vi "CalibrationManagementDemo.vi"() -> ()   [LabVIEW 2019]
uses:
  TypeDef/SlugExpiration.ctl
  ByteQXAPIBase/ByteQXAPIBase.lvclass
  TypeDef/CalibrationStates.ctl
  ByteQXAPIBase/FetchCalibration/Converted_Slug_Cluster.ctl
  ByteQXAPIBase/Instruments/Instrument.ctl
  ByteQXAPIBase/CalibrationMeasurements/CalibMeasure.ctl
  aa47c742-c095-4670-bf1f-6b28e4309cef.vi
  <vilib>/numeric/Random Number (Range) I64.vi
  <vilib>/Array/Sort 2D Array - Pop Stack.vi
  <vilib>/Array/Sort 2D Array - Push Stack.vi
  <vilib>/numeric/sub_Random U32.vi
panel:
  in  "Exit":bool
  out "Calibrations":string
  out "Status":string
  out "Calibration n.":string
  in  "Cancel":bool
  in  "Approvation":bool
  in  "Avanti":bool
  in  "Repeat":bool
  out "Outcome":string
  out "Measured value":dbl
  out "Reference value":dbl
  out "Waveform Chart":i64(graph)
  in  "Start Calibration":bool
  in  "Next":bool
  in  "Previus":bool
  out "Calibration n.":string
  in  "Filter":enum16{"All", "Expired", "Not Expired"}(ring)
  in  "Slug list":T1[](array[typedef])
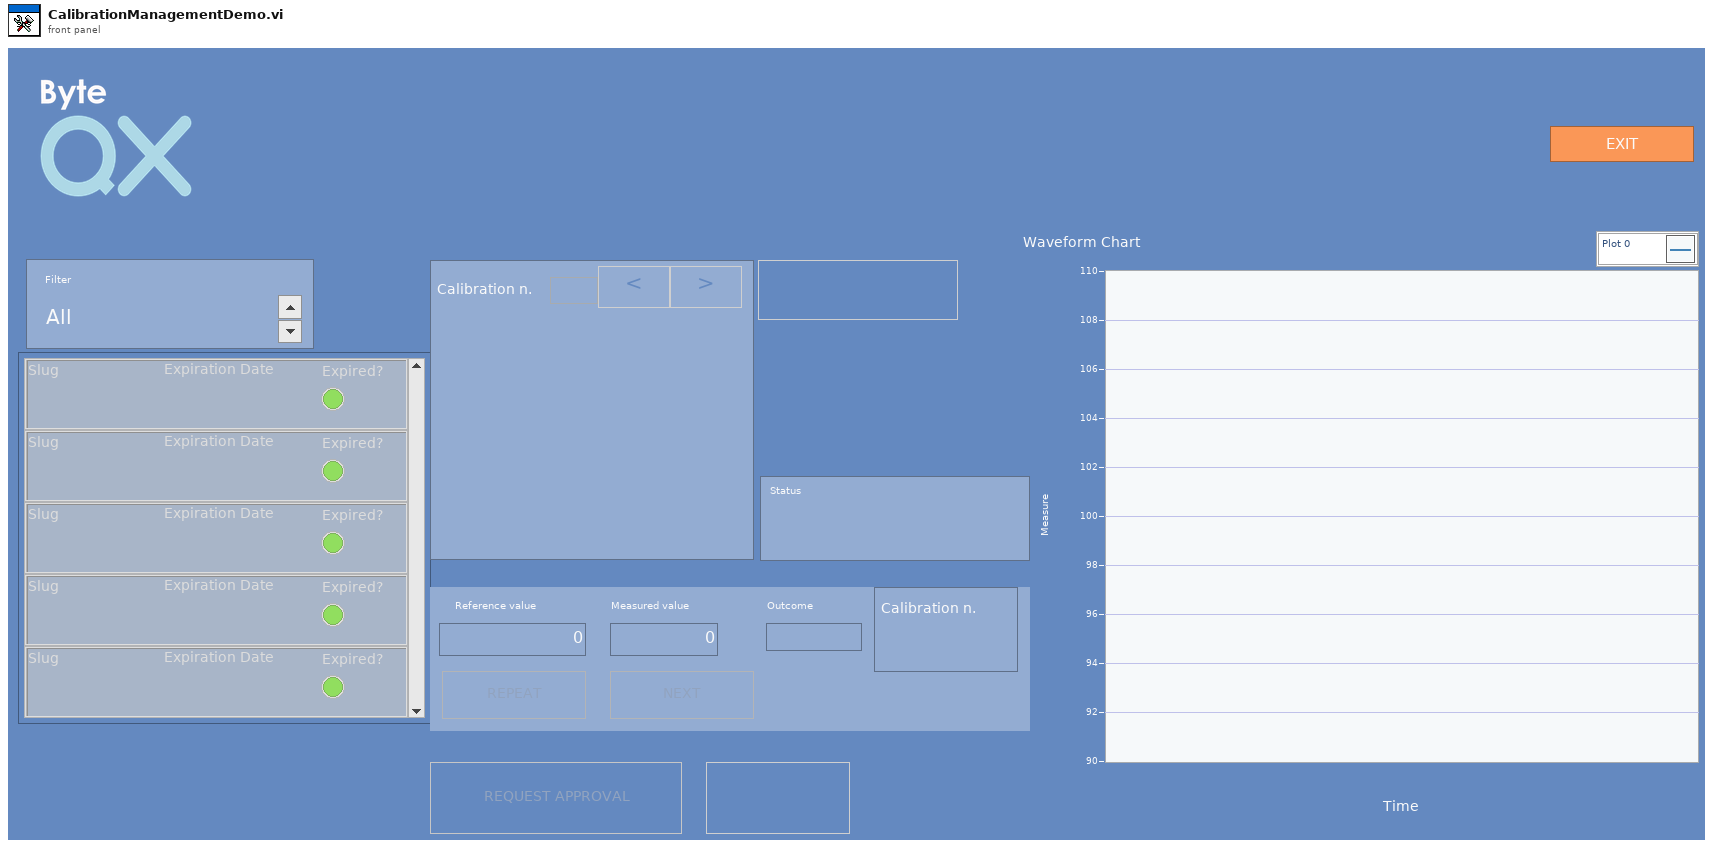
[diagram p1: front panel]
types:
  T1 = typedef "SlugExpiration.ctl" = cluster{"Slug":string, "Expiration Date":string, "Expired?":bool, "Id":i32, "active":bool, "Color Box":u32}
  T2 = typedef "CalibrationStates.ctl" = enum16{"Init", "Idle", "GetInstruments", "Fetch", "GetCalibrations", "CheckTotalMisurations", "StartCalibration", "ManageCalibration", "AllowApprove", "Approve"}
  T3 = typedef "ByteQXWebAPI.lvlib/ByteQXAPIBase.lvclass/CalibMeasure.ctl" = cluster{"controls":cluster{"id":u16, "descrizione":string, "numero_misure_necessarie":u16, "riferimento_obiettivo":dbl, "mpe_max":dbl, "mpe_min":dbl, "deviazione_standard":dbl, "incertezza":dbl, "numero_misure_effettuate":u32, "temperatura_c":dbl, "umidita":dbl, "strumento_riferimento":cluster{"id":u16, "nome":string}[]}[]}
  T4 = typedef "ByteQXWebAPI.lvlib/ByteQXAPIBase.lvclass/Instrument.ctl" = cluster{"id":i32, "slug":string, "stabilimento":cluster{"id":dbl}, "categoria":cluster{"id":dbl}, "tipologia_di_visualizzazione":cluster{"id":dbl}, "stato":cluster{"id":dbl}, "descrizione":string, "costruttore":string, "matricola":string, "data_registrazione":string, "intervallo_di_taratura_mesi":dbl, "reparto":string, "campo_misura":string, "risoluzione":dbl, "responsabile_strumento":string, "classe_di_precisione":string, "classificazione":string, "appunti":string, "manuale":string, "foto":string, "riferimento":bool, "qr_hashcode":string, "costo_euro":dbl}
  T5 = typedef "ByteQXWebAPI.lvlib/ByteQXAPIBase.lvclass/Converted_Slug_Cluster.ctl" = cluster{"id":u32, "instrument":string, "name":string, "date":timestamp}
  T6 = cluster{"Outcome":refnum<vi>, "Avanti":refnum<vi>, "Repeat":refnum<vi>, "Slug list":refnum<vi>, "Start Calibration":refnum<vi>, "Avanti":refnum<vi>, "Cancel":refnum<vi>, "Approvation":refnum<vi>}
  T7 = cluster{"ByteQXAPIBase in":refnum<class "ByteQXAPIBase.lvclass">, "Instruments_Slug":string[], "All_Instruments_Cals":T5[], "All_Instruments":T4[], "Slug list All":T1[], "Calibrations":T3, "Selected Slug":i32, "Misurazioni":string, "Misurazioni index":i32, "Next State":T2, "Waveform Chart":refnum<vi>, "New Val":dbl, "Id Failed":u32, "Failed?":bool, "Cal Index":i32, "Misurazioni n":string, "Stato":string, "Esito":string, "Misure effettuate":i32, "Calibrations":string}
  T8 = typedef "SlugExpiration1.ctl" = cluster{"Slug":string, "Expiration Date":string, "Expired?":bool, "Id":i32, "active":bool, "Color Box":u32}
  T9 = cluster{"id":u16, "descrizione":string, "numero_misure_necessarie":u16, "riferimento_obiettivo":dbl, "mpe_max":dbl, "mpe_min":dbl, "deviazione_standard":dbl, "incertezza":dbl, "numero_misure_effettuate":u32, "temperatura_c":dbl, "umidita":dbl, "strumento_riferimento":cluster{"id":u16, "nome":string}[]}[]
  T10 = cluster{"id":u16, "descrizione":string, "numero_misure_necessarie":u16, "riferimento_obiettivo":dbl, "mpe_max":dbl, "mpe_min":dbl, "deviazione_standard":dbl, "incertezza":dbl, "numero_misure_effettuate":u32, "temperatura_c":dbl, "umidita":dbl, "strumento_riferimento":cluster{"id":u16, "nome":string}[]}
  T11 = typedef "ByteQXWebAPI.lvlib/ByteQXAPIBase.lvclass/MeasurementResData.ctl" = cluster{"id":i32, "gruppo_misurazione":cluster{"id":i32}, "misura_strumento":dbl, "misura_riferimento":dbl, "is_correct":bool}
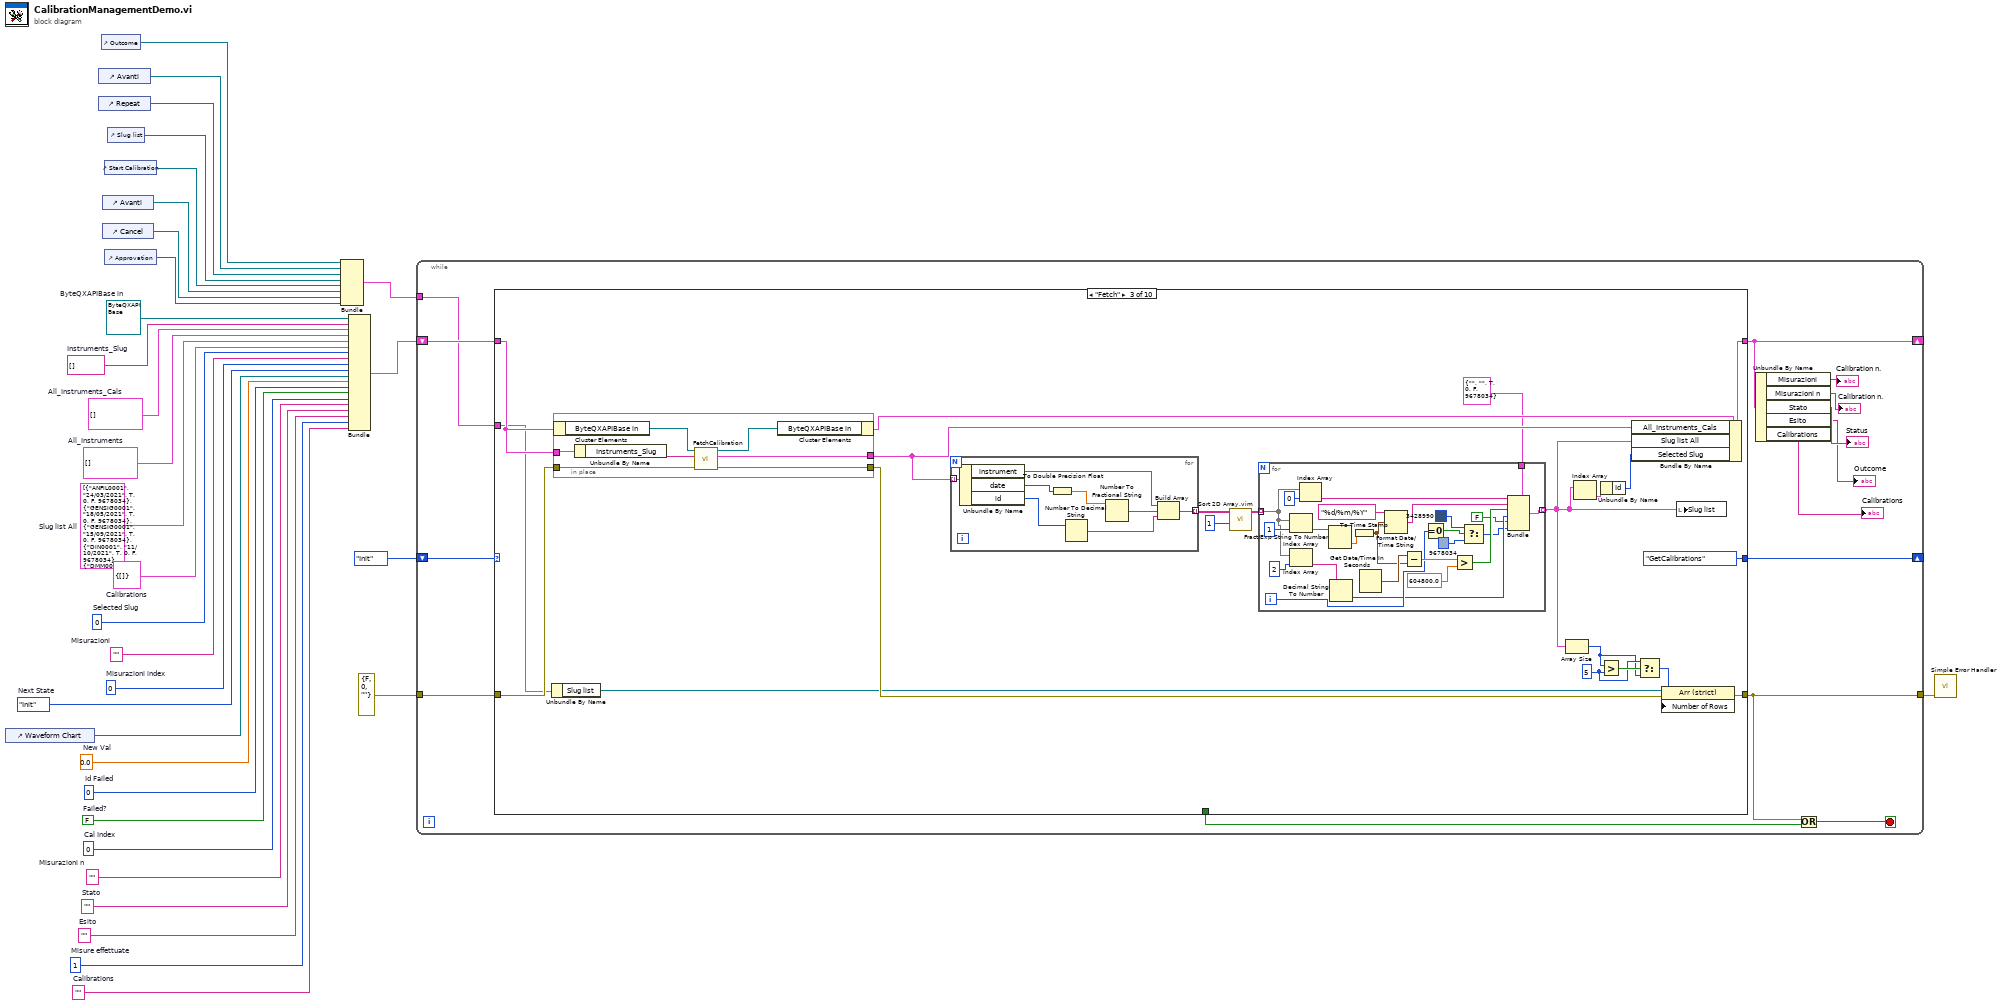
[diagram p0: block diagram]
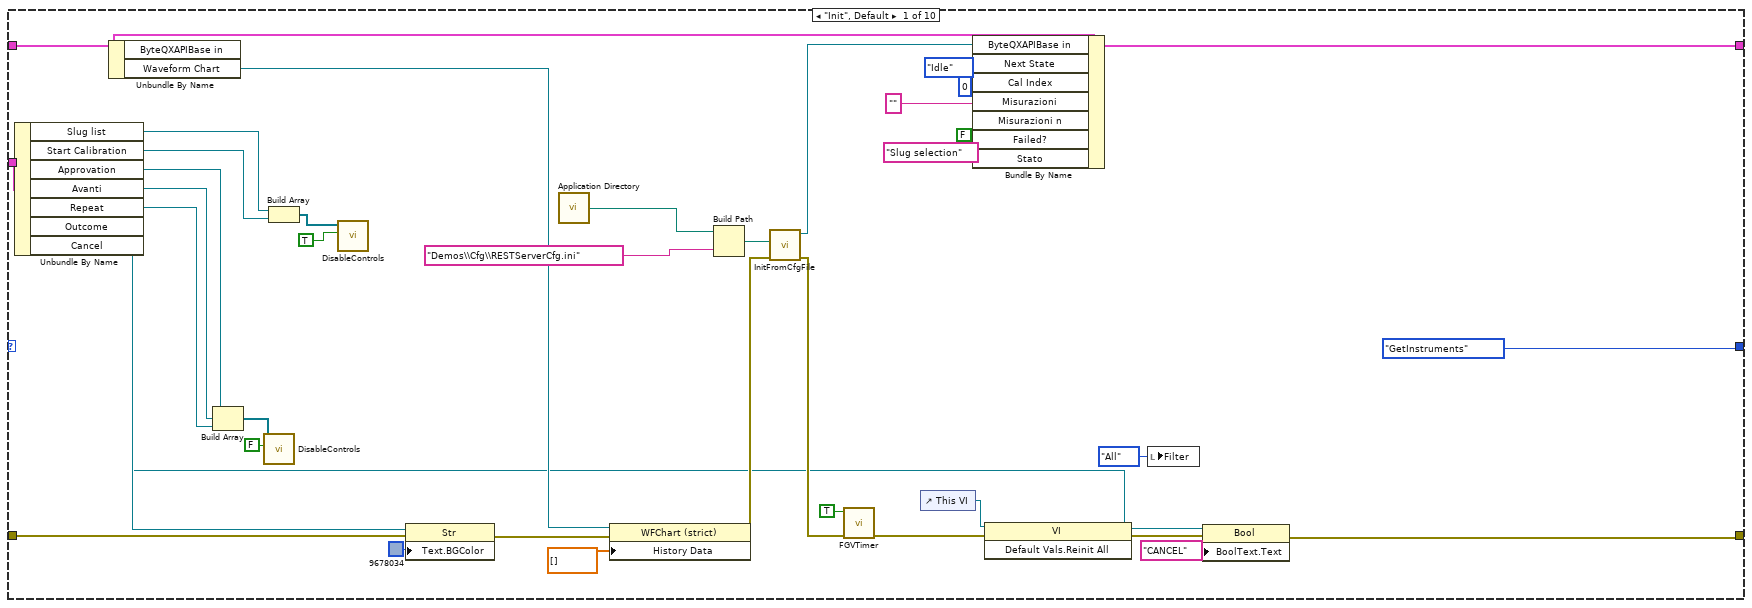
[diagram p2: hidden frame]
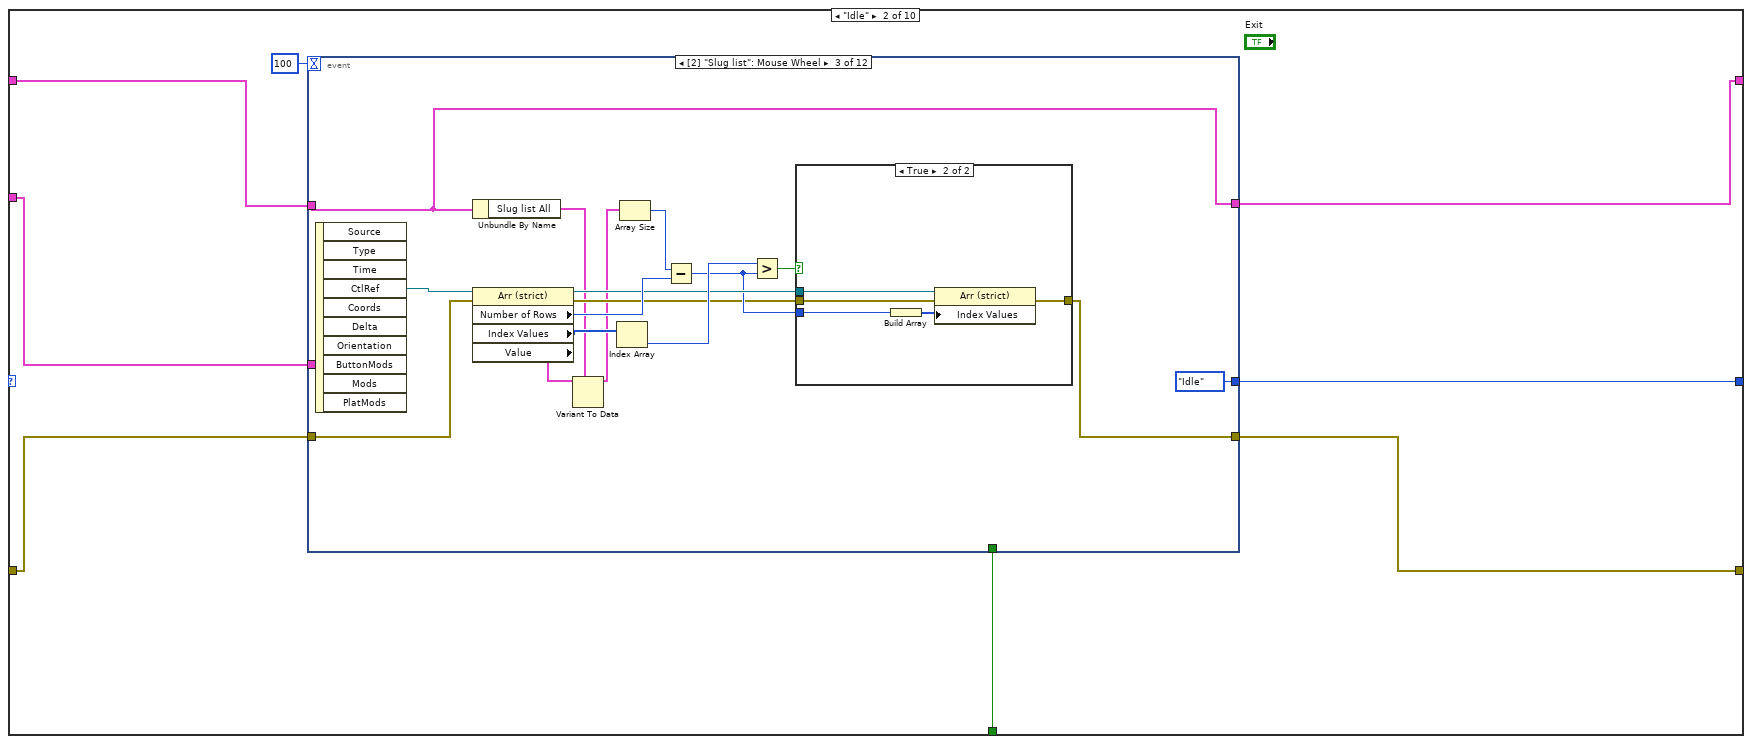
[diagram p3: hidden frame]
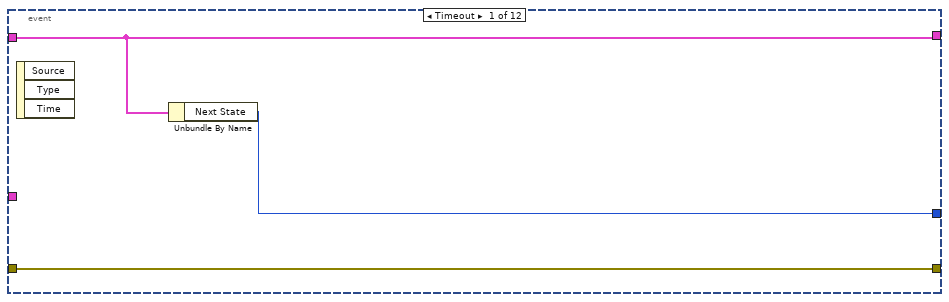
[diagram p4: hidden frame]
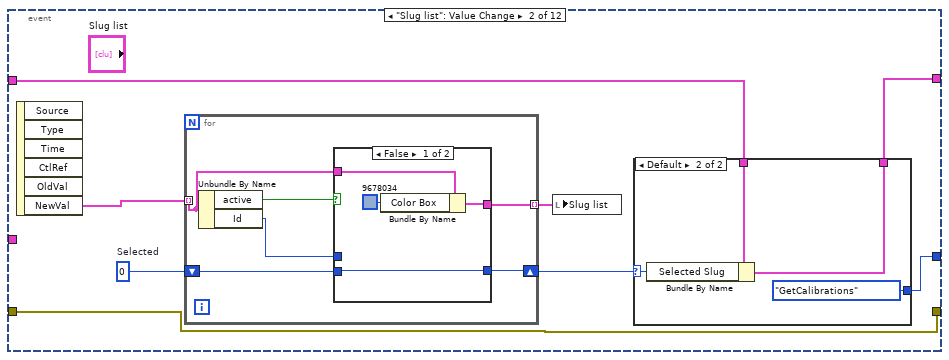
[diagram p5: hidden frame]
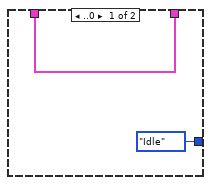
[diagram p6: hidden frame]
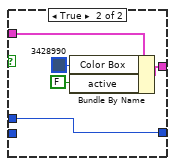
[diagram p7: hidden frame]
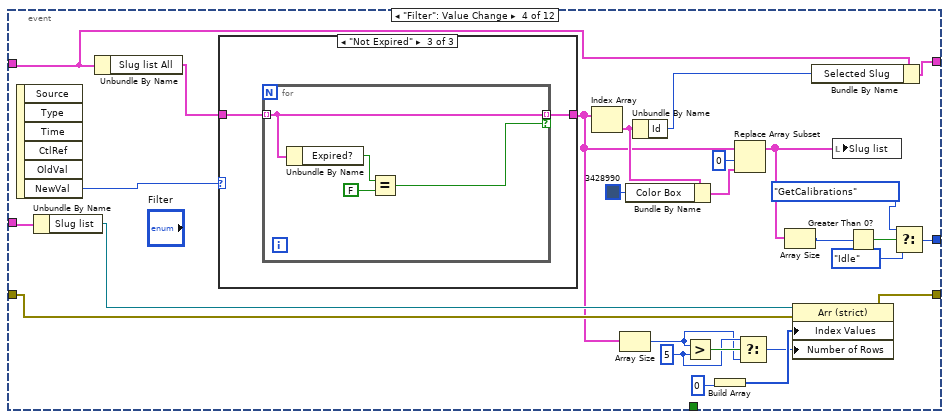
[diagram p9: hidden frame]
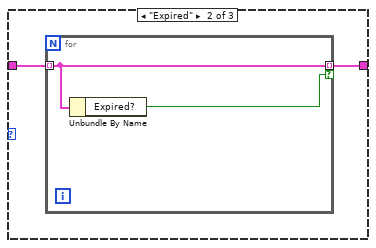
[diagram p11: hidden frame]
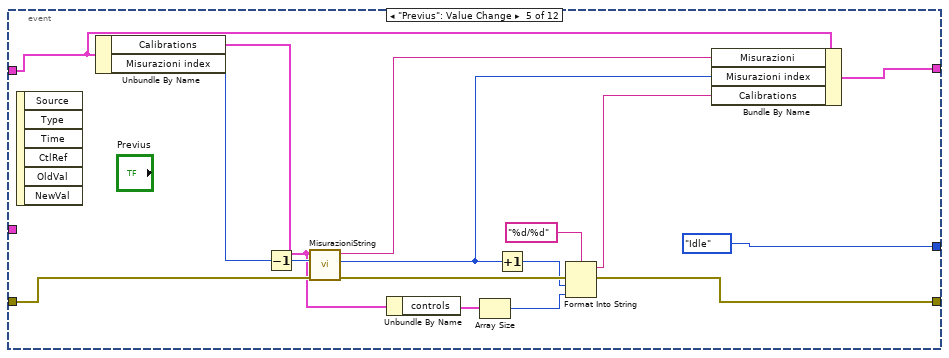
[diagram p12: hidden frame]
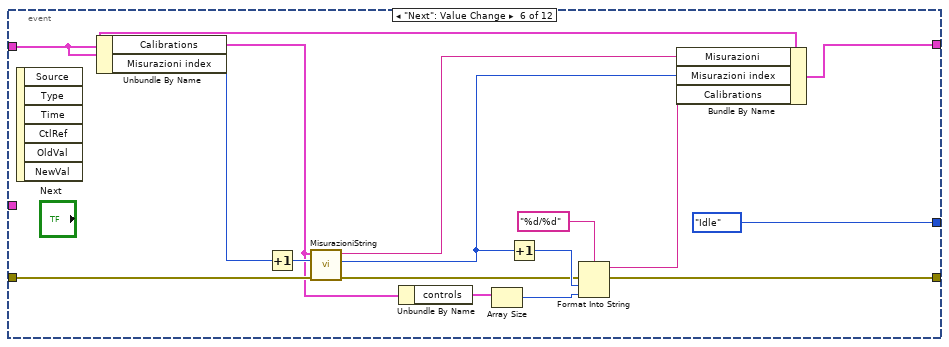
[diagram p13: hidden frame]
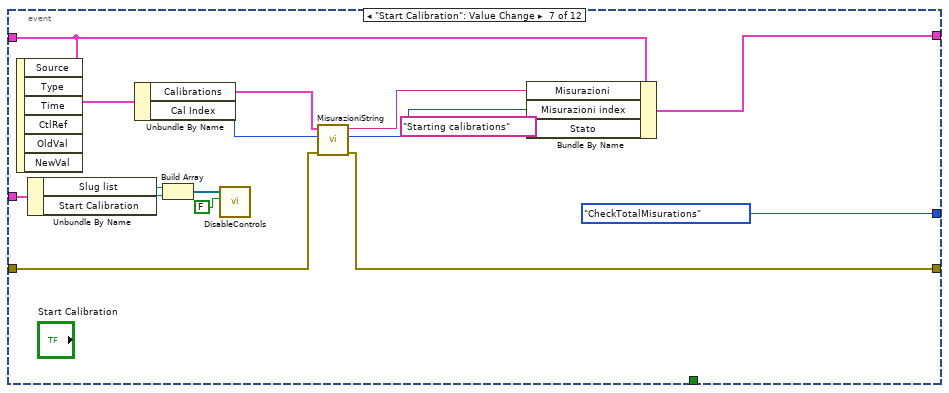
[diagram p14: hidden frame]
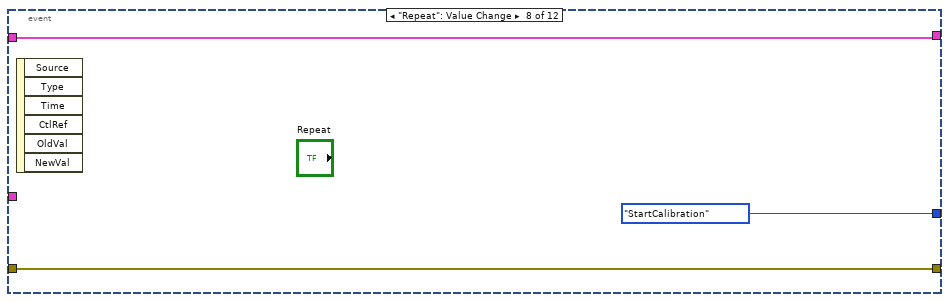
[diagram p15: hidden frame]
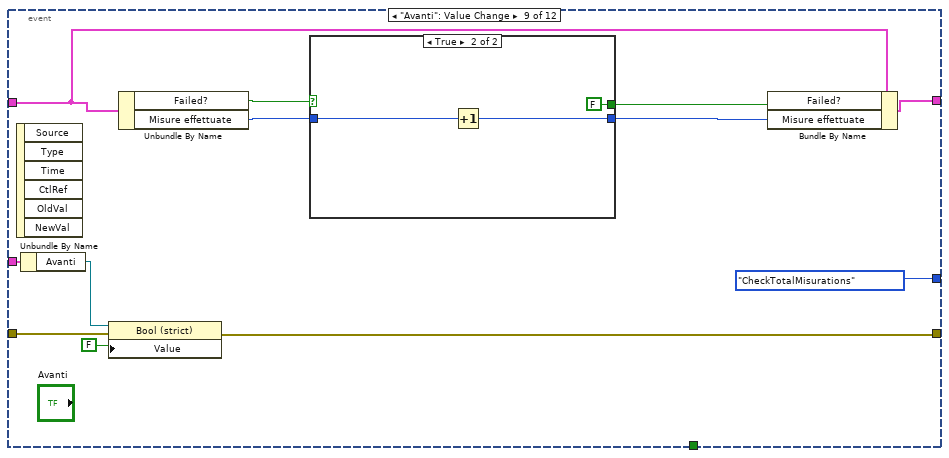
[diagram p16: hidden frame]
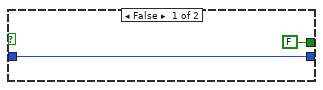
[diagram p17: hidden frame]
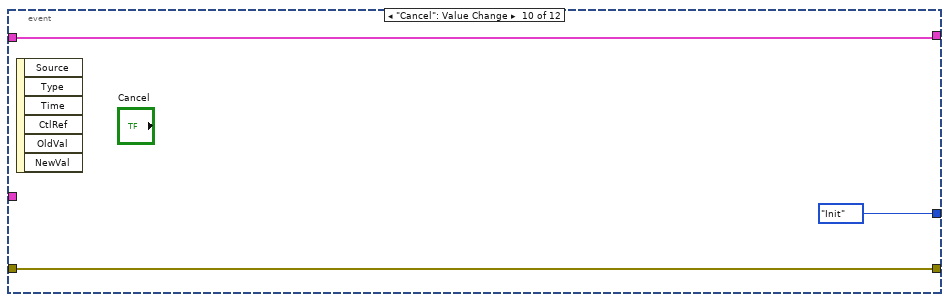
[diagram p18: hidden frame]
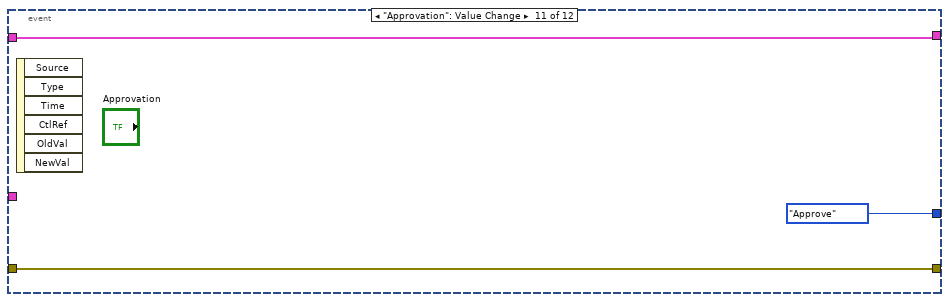
[diagram p19: hidden frame]
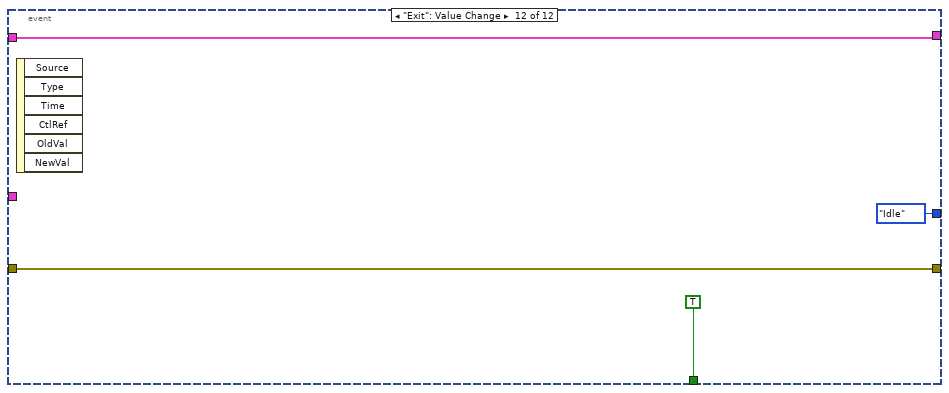
[diagram p20: hidden frame]
diagram:
  w2 = ""  # Calibrations
  w3 = 1  # Misure effettuate
  w5 = ""  # Esito
  w6 = ""  # Stato
  w11 = ""  # Misurazioni n
  w16 = 0  # Cal Index
  w17 = FALSE  # Failed?
  w18 = u32 0  # Id Failed
  w19 = 0.0  # New Val
  w21 = CalibrationStates."Init"  # Next State
  w22 = 0  # Misurazioni index
  w23 = ""  # Misurazioni
  w24 = T1[] [{"Slug"="ANFIL0001", "Expiration Date"="24/03/2021", "Expired?"=TRUE, "Id"=0, "active"=FALSE, "Color Box"=9678034}, {"Slug"="GENSIG0001", "Expiration Date"="18/05/2021", "Expired?"=TRUE, "Id"=0, "active"=FALSE, "Color Box"=9678034}, {"Slug"="GENSIG0001", "Expiration Date"="15/09/2021", "Expired?"=TRUE, "Id"=0, "active"=FALSE, "Color Box"=9678034}, {"Slug"="DIN0001", "Expiration Date"="11/10/2021", "Expired?"=TRUE, "Id"=0, "active"=FALSE, "Color Box"=9678034}, {"Slug"="DMM0002", "Expiration Date"="20/10/2021", "Expired?"=TRUE, "Id"=0, "active"=FALSE, "Color Box"=9678034}, {"Slug"="COMP0001", "Expiration Date"="01/12/2021", "Expired?"=TRUE, "Id"=0, "active"=FALSE, "Color Box"=9678034}, {"Slug"="TORS0002", "Expiration Date"="06/12/2021", "Expired?"=TRUE, "Id"=0, "active"=FALSE, "Color Box"=9678034}, {"Slug"="CDIND0001", "Expiration Date"="04/03/2022", "Expired?"=TRUE, "Id"=0, "active"=FALSE, "Color Box"=9678034}, {"Slug"="CALI0004", "Expiration Date"="11/03/2022", "Expired?"=TRUE, "Id"=0, "active"=FALSE, "Color Box"=9678034}, {"Slug"="CALI0001", "Expiration Date"="10/05/2022", "Expired?"=TRUE, "Id"=0, "active"=FALSE, "Color Box"=9678034}, {"Slug"="CALI0012", "Expiration Date"="10/05/2022", "Expired?"=TRUE, "Id"=0, "active"=FALSE, "Color Box"=9678034}, {"Slug"="CALI0011", "Expiration Date"="11/05/2022", "Expired?"=TRUE, "Id"=0, "active"=FALSE, "Color Box"=9678034}, {"Slug"="CALI0014", "Expiration Date"="04/07/2022", "Expired?"=TRUE, "Id"=0, "active"=FALSE, "Color Box"=9678034}, {"Slug"="CDIND0001", "Expiration Date"="15/07/2022", "Expired?"=TRUE, "Id"=0, "active"=FALSE, "Color Box"=9678034}, {"Slug"="CALI0024", "Expiration Date"="11/07/2023", "Expired?"=TRUE, "Id"=0, "active"=FALSE, "Color Box"=9678034}, {"Slug"="CALI0017", "Expiration Date"="19/09/2023", "Expired?"=TRUE, "Id"=0, "active"=FALSE, "Color Box"=9678034}, {"Slug"="CALI0020", "Expiration Date"="02/11/2023", "Expired?"=TRUE, "Id"=0, "active"=FALSE, "Color Box"=9678034}, {"Slug"="CALI0017", "Expiration Date"="03/11/2023", "Expired?"=TRUE, "Id"=0, "active"=FALSE, "Color Box"=9678034}, {"Slug"="CALI0025", "Expiration Date"="11/11/2023", "Expired?"=TRUE, "Id"=0, "active"=FALSE, "Color Box"=9678034}, {"Slug"="CLBR0001", "Expiration Date"="30/11/2023", "Expired?"=TRUE, "Id"=0, "active"=FALSE, "Color Box"=9678034}, {"Slug"="CLBR0001", "Expiration Date"="02/01/2024", "Expired?"=TRUE, "Id"=0, "active"=FALSE, "Color Box"=9678034}, {"Slug"="CLBR0001", "Expiration Date"="02/01/2024", "Expired?"=TRUE, "Id"=0, "active"=FALSE, "Color Box"=9678034}, {"Slug"="CLBR0003", "Expiration Date"="04/03/2024", "Expired?"=TRUE, "Id"=0, "active"=FALSE, "Color Box"=9678034}, {"Slug"="MICP0001", "Expiration Date"="19/03/2024", "Expired?"=TRUE, "Id"=0, "active"=FALSE, "Color Box"=9678034}, {"Slug"="TERM0002", "Expiration Date"="04/07/2024", "Expired?"=TRUE, "Id"=0, "active"=FALSE, "Color Box"=9678034}, {"Slug"="ACCEL0008", "Expiration Date"="04/07/2024", "Expired?"=TRUE, "Id"=0, "active"=FALSE, "Color Box"=9678034}, {"Slug"="ACCEL0008", "Expiration Date"="05/07/2024", "Expired?"=TRUE, "Id"=0, "active"=FALSE, "Color Box"=9678034}, {"Slug"="ACCEL0008", "Expiration Date"="19/08/2024", "Expired?"=TRUE, "Id"=0, "active"=FALSE, "Color Box"=9678034}, {"Slug"="TERM0002", "Expiration Date"="15/10/2024", "Expired?"=TRUE, "Id"=0, "active"=FALSE, "Color Box"=9678034}, {"Slug"="BILA0001", "Expiration Date"="15/10/2024", "Expired?"=TRUE, "Id"=0, "active"=FALSE, "Color Box"=9678034}, {"Slug"="CLBR0001", "Expiration Date"="15/10/2024", "Expired?"=TRUE, "Id"=0, "active"=FALSE, "Color Box"=9678034}, {"Slug"="ACCEL0002", "Expiration Date"="15/10/2024", "Expired?"=TRUE, "Id"=0, "active"=FALSE, "Color Box"=9678034}]  # Slug list All
  w25 = 0  # Selected Slug
  w26 = T3 {"controls"=[]}  # Calibrations
  w27 = T4[] []  # All_Instruments
  w28 = T5[] []  # All_Instruments_Cals
  w29 = string[] []  # Instruments_Slug
  w32 = refnum<class "ByteQXAPIBase.lvclass"> refnum  # ByteQXAPIBase in
  n1 = control-ref of="Waveform Chart"() -> (w20:refnum<vi>)
  n2 = control-ref of="Avanti"() -> (w7:refnum<vi>)
  n3 = control-ref of="Repeat"() -> (w8:refnum<vi>)
  n4 = control-ref of="Outcome"() -> (w4:refnum<vi>)
  n5 = control-ref of="Avanti"() -> (w12:refnum<vi>)
  n6 = control-ref of="Cancel"() -> (w13:refnum<vi>)
  n7 = control-ref of="Start Calibration"() -> (w10:refnum<vi>)
  n8 = control-ref of="Approvation"() -> (w14:refnum<vi>)
  n9 = control-ref of="Slug list"() -> (w9:refnum<vi>)
  n10 = Bundle("Outcome"=w4, "Avanti"=w7, "Repeat"=w8, "Slug list"=w9, "Start Calibration"=w10, "Avanti"=w12, "Cancel"=w13, "Approvation"=w14) -> (w15:T6)  [unwired: 1 in]
  n11 = Bundle("ByteQXAPIBase in"=w32, "Instruments_Slug"=w29, "All_Instruments_Cals"=w28, "All_Instruments"=w27, "Slug list All"=w24, "Calibrations"=w26, "Selected Slug"=w25, "Misurazioni"=w23, "Misurazioni index"=w22, "Next State"=w21, "Waveform Chart"=w20, "New Val"=w19, "Id Failed"=w18, "Failed?"=w17, "Cal Index"=w16, "Misurazioni n"=w11, "Stato"=w6, "Esito"=w5, "Misure effettuate"=w3, "Calibrations"=w2) -> (w31:T7)  [unwired: 1 in]
  n12 = while {
    shift-right: [w46] -> _
    shift-left: CalibrationStates."Init" -> [w47]
    shift-right: [w43] -> _
    shift-left: w31 -> [w45]
    tunnel: w15 -> [w41]
    tunnel: errorcluster {"status"=FALSE, "code"=0, "source"=""} ("error in (no error)") -> [w44]
    tunnel: [w34] -> w1
    stop <- w36 stop-if-true
    n13 = case shown="\"Fetch\"" w47 {
      tunnel: [CalibrationStates."GetInstruments" w91 CalibrationStates."GetCalibrations" CalibrationStates."Fetch" CalibrationStates."Idle" w376 CalibrationStates."Idle" CalibrationStates."Idle" CalibrationStates."Idle" CalibrationStates."Idle"] -> w46
      tunnel: w45 -> [w82 w93 w282 w328 w357 w372 w448 w484 w550 w587]
      tunnel: w44 -> [w54 w90 w281 w330 w358 w374 w433 w471 w553 w586]
      tunnel: [w49 w89 w269 w324 w350 w373 w423 w472 w553 w575] -> w34
      tunnel: [w80 w92 w278 w326 w356 w371 w447 w483 w550 w579] -> w43
      tunnel: w41 -> [w70 w87 w270 _ w343 w375 w437 w477 w559 w584]
      tunnel: [_ w86 _ _ _ _ _ _ _ _] -> w35
      frame "Init", Default {
        w67 = "" ("Misurazioni")
        n14 = Unbundle By Name(w70) -> ("Slug list"=w66:refnum<vi>, "Start Calibration"=w65:refnum<vi>, "Approvation"=w48:refnum<vi>, "Avanti"=w60:refnum<vi>, "Repeat"=w59:refnum<vi>, "Outcome"=w53:refnum<vi>, "Cancel"=w51:refnum<vi>)
        n15 = Unbundle By Name(w82) -> ("Waveform Chart"=w74:refnum<vi>)  [unwired: 1 out]
        n16 = Build Array(w48, w60, w59) -> (w62:refnum<vi>[])
        n17 = call "DisableControls.vi"("Visible"=FALSE, "Controls"=w62) -> ()  [unwired: 9 in, 1 out]
        n18 = Build Array(w66, w65) -> (w64:refnum<vi>[])
        n19 = call "DisableControls.vi"("Visible"=TRUE, "Controls"=w64) -> ()  [unwired: 9 in, 1 out]
        n20 = property class="Str"(reference=w53, error in=w54, "Text.BGColor"=u32 9678034 ("Text.Text Colors:BG Color")) -> (error out=w55:errorcluster)  [unwired: 1 out]
        n21 = call <vilib>:"Application Directory.vi"() -> ("Application Directory"=w83:path)
        n22 = property class="WFChart (strict)"(reference=w74, error in=w55, "History Data"=dbl[] []) -> (error out=w73:errorcluster)  [unwired: 1 out]
        n23 = Build Path(base path=w83, name or relative path="Demos\\Cfg\\RESTServerCfg.ini") -> (appended path=w79:path)
        n24 = call "InitFromCfgFile.vi"("error in (no error)"=w73, "configuration file path"=w79) -> ("error out"=w77:errorcluster, "ByteQXAPIBase out"=w81:refnum<class "ByteQXAPIBase.lvclass">)  [unwired: 8 in]
        n25 = call "FGVTimer.vi"("error in"=w77, "Reset"=TRUE) -> ("error out"=w69:errorcluster)  [unwired: 7 in, 2 out]
        n26 = control-ref of="This VI"() -> (w68:refnum<vi>)
        n27 = Bundle By Name(cluster=w82, "ByteQXAPIBase in"=w81, "Next State"=CalibrationStates."Idle", "Cal Index"=0, "Misurazioni"=w67, "Misurazioni n"=w67, "Failed?"=FALSE, "Stato"="Slug selection") -> (w80:T7)
        n28 = invoke class="VI" method="Default Vals.Reinit All"(reference=w68, error in=w69) -> (error out=w52:errorcluster)  [unwired: 1 in, 2 out]
        n29 = local write "Filter"(enum16{"All", "Expired", "Not Expired"}."All" ("Filter")) -> ()
        n30 = property class="Bool"(reference=w51, error in=w52, "BoolText.Text"="CANCEL" ("Boolean Text.Text")) -> (error out=w49:errorcluster)  [unwired: 1 out]
      }
      frame "Idle" {
        n31 = event shown="[2] \"Slug list\": Mouse Wheel" {
          selector: _ -> [_ _ _ _ _ _ _ _ _ _ _ _]
          dyn-events: _ -> [_ _ _ _ _ _ _ _ _ _ _ _]
          timeout: 100 -> [_ _ _ _ _ _ _ _ _ _ _ _]
          tunnel: w93 -> [w95 w101 w129 w171 w197 w213 w228 w234 w238 w252 w255 w258]
          tunnel: [w95 w99 w129 w170 w196 w211 w225 w234 w237 w252 w255 w258] -> w92
          tunnel: [w94 w98 CalibrationStates."Idle" w148 CalibrationStates."Idle" CalibrationStates."Idle" CalibrationStates."CheckTotalMisurations" CalibrationStates."StartCalibration" CalibrationStates."CheckTotalMisurations" CalibrationStates."Init" CalibrationStates."Approve" CalibrationStates."Idle"] -> w91
          tunnel: w90 -> [w96 w97 w133 w161 w194 w216 w224 w232 w241 w254 w257 w260]
          tunnel: [w96 w97 w131 w160 w192 w202 w222 w232 w242 w254 w257 w260] -> w89
          tunnel: w87 -> [_ _ _ w163 _ _ w223 _ w243 _ _ _]
          tunnel: [_ _ _ _ _ _ _ _ _ _ _ TRUE] -> w86
          event Timeout {
            n32 = event-data() -> ()  [unwired: 1 in, 3 out]
            n33 = Unbundle By Name(w95) -> ("Next State"=w94:T2)
          }
          event "Slug list": Value Change {
            w102 = 0  # Selected
            n34 = event-data() -> ("NewVal"=w104:T1[])  [unwired: 1 in, 5 out]
            n35 = for {
              tunnel: w104 -> [w116] mode=indexing
              tunnel: [w115] -> w103 mode=indexing
              shift-right: [w113] -> w100
              shift-left: w102 -> [w114]
              n36 = Unbundle By Name(w116) -> ("active"=w111:bool, "Id"=w112:i32)
              n37 = case shown="False" w111 {
                tunnel: w116 -> [w119 w125]
                tunnel: [w120 w123] -> w115
                tunnel: w114 -> [w117 _]
                tunnel: [w117 w121] -> w113
                tunnel: w112 -> [_ w121]
                frame False {
                  n38 = Bundle By Name(cluster=w119, "Color Box"=u32 9678034) -> (w120:T1)
                }
                frame True {
                  n39 = Bundle By Name(cluster=w125, "Color Box"=u32 3428990, "active"=FALSE ("Active")) -> (w123:T1)
                }
              }
            }
            n40 = local write "Slug list"(w103) -> ()
            n41 = case shown="Default" w100 {
              selector: w100 -> [_ w109]
              tunnel: w101 -> [w106 w110]
              tunnel: [w106 w108] -> w99
              tunnel: [CalibrationStates."Idle" CalibrationStates."GetCalibrations"] -> w98
              frame ..0 {
              }
              frame Default {
                n42 = Bundle By Name(cluster=w110, "Selected Slug"=w109) -> (w108:T7)
              }
            }
          }
          event "Slug list": Mouse Wheel {
            n43 = event-data() -> ("CtlRef"=w141:refnum<vi>)  [unwired: 1 in, 9 out]
            n44 = Unbundle By Name(w129) -> ("Slug list All"=w126:T1[])
            n45 = property class="Arr (strict)"(reference=w141, error in=w133) -> (reference out=w135:refnum<vi>, error out=w132:errorcluster, "Number of Rows"=w138:u32, "Index Values"=w140:u32[], "Value"=w127:T8[])
            n46 = Variant To Data(type=w126, Variant=w127) -> (data=w128:T1[])  [unwired: 1 in, 1 out]
            n47 = Index Array(array=w140) -> (element=w137:u32)  [unwired: 1 in]
            n48 = Array Size(array=w128) -> (size(s)=w139:i32)
            n49 = Subtract(x=w139, y=w138) -> (x-y=w134:u32)
            n50 = Greater?(x=w137, y=w134) -> (0:w136:bool)
            n51 = case shown="True" w136 {
              tunnel: w135 -> [_ w147]
              tunnel: w134 -> [_ w146]
              tunnel: w132 -> [w142 w144]
              tunnel: [w142 w143] -> w131
              frame False {
              }
              frame True {
                n52 = Build Array(w146) -> (w145:u32[])
                n53 = property class="Arr (strict)"(reference=w147, error in=w144, "Index Values"=w145) -> (error out=w143:errorcluster)  [unwired: 1 out]
              }
            }
          }
          event "Filter": Value Change {
            w157 = 5 ("y")
            n54 = event-data() -> ("NewVal"=w173:enum16{"All", "Expired", "Not Expired"})  [unwired: 1 in, 5 out]
            n55 = Unbundle By Name(w163) -> ("Slug list"=w162:refnum<vi>)
            n56 = Unbundle By Name(w171) -> ("Slug list All"=w172:T1[])
            n57 = case shown="\"Not Expired\"" w173 {
              tunnel: w172 -> [w174 w176 w180]
              tunnel: [w174 w175 w179] -> w154
              frame "All" {
              }
              frame "Expired" {
                n58 = for {
                  tunnel: w176 -> [w178] mode=indexing
                  tunnel: [w178] -> w175 mode=indexing if=w177
                  n59 = Unbundle By Name(w178) -> ("Expired?"=w177:bool)
                }
              }
              frame "Not Expired" {
                n60 = for {
                  tunnel: w180 -> [w184] mode=indexing
                  tunnel: [w184] -> w179 mode=indexing if=w181
                  n61 = Unbundle By Name(w184) -> ("Expired?"=w183:bool)
                  n62 = Equal?(x=w183, y=FALSE) -> (x = y?=w181:bool)
                }
              }
            }
            n63 = Index Array(array=w154) -> (element=w168:T1)  [unwired: 1 in]
            n64 = Array Size(array=w154) -> (size(s)=w156:i32)
            n65 = Bundle By Name(cluster=w168, "Color Box"=u32 3428990) -> (w166:T1)
            n66 = Unbundle By Name(w168) -> ("Id"=w169:i32)
            n67 = Greater?(x=w156, y=w157) -> (0:w158:bool)
            n68 = Build Array(0) -> (w164:i32[])
            n69 = Replace Array Subset(array=w154, new element=w166, index=0) -> (w151:T1[])
            n70 = Select(t=w157, s=w158, f=w156) -> (s? t:f=w155:i32)
            n71 = Array Size(array=w151) -> (size(s)=w152:i32)
            n72 = property class="Arr (strict)"(reference=w162, error in=w161, "Index Values"=w164, "Number of Rows"=w155) -> (error out=w160:errorcluster)  [unwired: 1 out]
            n73 = Bundle By Name(cluster=w171, "Selected Slug"=w169) -> (w170:T7)
            n74 = local write "Slug list"(w151) -> ()
            n75 = Greater Than 0?(x=w152) -> (x > 0?=w153:bool)
            n76 = Select(t=CalibrationStates."GetCalibrations", s=w153, f=CalibrationStates."Idle") -> (s? t:f=w148:T2)
          }
          event "Previus": Value Change {
            n77 = event-data() -> ()  [unwired: 1 in, 6 out]
            n78 = Unbundle By Name(w197) -> ("Calibrations"=w188:T3, "Misurazioni index"=w199:i32)
            n79 = Decrement(x=w199) -> (x-1=w200:i32)
            n80 = call "MisurazioniString.vi"("error in (no error)"=w194, "index"=w200, "Calibration data"=w188) -> ("error out"=w193:errorcluster, "index"=w190:i32, "String"=w198:string)  [unwired: 6 in]
            n81 = Unbundle By Name(w188) -> ("controls"=w187:T9)
            n82 = Array Size(array=w187) -> (size(s)=w186:i32)
            n83 = Increment(x=w190) -> (x+1=w189:i32)
            n84 = Format Into String(format string="%d/%d", error in=w193, w189, w186) -> (resulting string=w185:string, error out=w192:errorcluster)  [unwired: 1 in]
            n85 = Bundle By Name(cluster=w197, "Misurazioni"=w198, "Misurazioni index"=w190, "Calibrations"=w185) -> (w196:T7)
          }
          event "Next": Value Change {
            n86 = event-data() -> ()  [unwired: 1 in, 6 out]
            n87 = Unbundle By Name(w213) -> ("Calibrations"=w207:T3, "Misurazioni index"=w214:i32)
            n88 = Increment(x=w214) -> (x+1=w215:i32)
            n89 = call "MisurazioniString.vi"("error in (no error)"=w216, "index"=w215, "Calibration data"=w207) -> ("error out"=w205:errorcluster, "index"=w204:i32, "String"=w212:string)  [unwired: 6 in]
            n90 = Unbundle By Name(w207) -> ("controls"=w203:T9)
            n91 = Array Size(array=w203) -> (size(s)=w206:i32)
            n92 = Increment(x=w204) -> (x+1=w208:i32)
            n93 = Format Into String(format string="%d/%d", error in=w205, w208, w206) -> (resulting string=w201:string, error out=w202:errorcluster)  [unwired: 1 in]
            n94 = Bundle By Name(cluster=w213, "Misurazioni"=w212, "Misurazioni index"=w204, "Calibrations"=w201) -> (w211:T7)
          }
          event "Start Calibration": Value Change {
            n95 = event-data() -> ()  [unwired: 1 in, 6 out]
            n96 = Unbundle By Name(w223) -> ("Slug list"=w221:refnum<vi>, "Start Calibration"=w220:refnum<vi>)
            n97 = Unbundle By Name(w228) -> ("Calibrations"=w230:T3, "Cal Index"=w229:i32)
            n98 = Build Array(w221, w220) -> (w219:refnum<vi>[])
            n99 = call "DisableControls.vi"("Visible"=FALSE, "Controls"=w219) -> ()  [unwired: 9 in, 1 out]
            n100 = call "MisurazioniString.vi"("error in (no error)"=w224, "index"=w229, "Calibration data"=w230) -> ("error out"=w222:errorcluster, "index"=w226:i32, "String"=w227:string)  [unwired: 6 in]
            n101 = Bundle By Name(cluster=w228, "Misurazioni"=w227, "Misurazioni index"=w226, "Stato"="Starting calibrations") -> (w225:T7)
          }
          event "Repeat": Value Change {
            n102 = event-data() -> ()  [unwired: 1 in, 6 out]
          }
          event "Avanti": Value Change {
            n103 = event-data() -> ()  [unwired: 1 in, 6 out]
            n104 = Unbundle By Name(w243) -> ("Avanti"=w245:refnum<vi>)
            n105 = property class="Bool (strict)"(reference=w245, error in=w241, "Value"=FALSE) -> (error out=w242:errorcluster)  [unwired: 1 out]
            n106 = Unbundle By Name(w238) -> ("Failed?"=w240:bool, "Misure effettuate"=w239:i32)
            n107 = case shown="True" w240 {
              tunnel: w239 -> [w248 w251]
              tunnel: [w248 w250] -> w236
              tunnel: [FALSE FALSE] -> w235
              frame False {
              }
              frame True {
                n108 = Increment(x=w251) -> (x+1=w250:i32)
              }
            }
            n109 = Bundle By Name(cluster=w238, "Failed?"=w235, "Misure effettuate"=w236) -> (w237:T7)
          }
          event "Cancel": Value Change {
            n110 = event-data() -> ()  [unwired: 1 in, 6 out]
          }
          event "Approvation": Value Change {
            n111 = event-data() -> ()  [unwired: 1 in, 6 out]
          }
          event "Exit": Value Change {
            n112 = event-data() -> ()  [unwired: 1 in, 6 out]
          }
        }
      }
      frame "Fetch" {
        w265 = 5 ("y")
        n113 = Unbundle By Name(w270) -> ("Slug list"=w267:refnum<vi>)
        n114 = in-place {
          in-place-border: w281 -> [w320]
          in-place-border: [w319] -> w268
          in-place-border: [w318] -> w274
          in-place-border: w282 -> [w316]
          n115 = in-place-cluster #1(w282) -> ("ByteQXAPIBase in"=w317:refnum<class "ByteQXAPIBase.lvclass">)
          n116 = Unbundle By Name(w316) -> ("Instruments_Slug"=w315:string[])
          n117 = call-dynamic "FetchCalibration.vi"("error in (no error)"=w320, "instruments"=w315, "ByteQXAPIBase in"=w317) -> ("error out"=w319:errorcluster, "instruments"=w318:T5[], "ByteQXAPIBase out"=w321:refnum<class "ByteQXAPIBase.lvclass">)  [unwired: 6 in]
          n118 = in-place-cluster #1("ByteQXAPIBase in"=w321) -> (w279:T7)
        }
        n119 = for {
          tunnel: w274 -> [w314] mode=indexing
          tunnel: [w313] -> w277 mode=indexing
          n120 = Unbundle By Name(w314) -> ("instrument"=w312:string, "date"=w311:timestamp, "id"=w308:u32)
          n121 = To Double Precision Float(number=w311) -> (double precision float=w310:dbl)
          n122 = Number To Decimal String(number=w308) -> (decimal integer string=w307:string)  [unwired: 1 in]
          n123 = Number To Fractional String(number=w310) -> (F-format string=w309:string)  [unwired: 3 in]
          n124 = Build Array(w312, w309, w307) -> (w313:string[])
        }
        n125 = call "Sort 2D Array.vim"("index"=1, "2D array"=w277) -> ("sorted 2D array"=w275:string[][])  [unwired: 8 in, 1 out]
        n126 = for {
          tunnel: w275 -> [w292] mode=indexing
          tunnel: T1 {"Slug"="", "Expiration Date"="", "Expired?"=TRUE, "Id"=0, "active"=FALSE, "Color Box"=9678034} ("Slug list") -> [w306]
          tunnel: [w298] -> w262 mode=indexing
          i -> [w290]
          n127 = Index Array(array=w292, index=1) -> (element=w302:string)
          n128 = Index Array(array=w292, index=2) -> (element=w291:string)
          n129 = Index Array(array=w292, index=0) -> (element=w304:string)
          n130 = Fract/Exp String To Number(string=w302) -> (number=w301:dbl)  [unwired: 3 in, 1 out]
          n131 = Decimal String To Number(string=w291) -> (number=w285:i32)  [unwired: 2 in, 1 out]
          n132 = To Time Stamp(1:w301) -> (0:w294:timestamp)
          n133 = Get Date/Time In Seconds() -> (seconds since 1Jan1904=w295:timestamp)
          n134 = Format Date/Time String(time format string (%c)="%d/%m/%Y", seconds (now)=w294) -> (date/time string=w299:string)  [unwired: 1 in]
          n135 = Subtract(x=w295, y=w294) -> (x-y=w297:dbl)
          n136 = Equal To 0?(x=w290) -> (x = 0?=w289:bool)
          n137 = Greater?(x=w297, y=604800.0) -> (0:w286:bool)
          n138 = Select(t=u32 3428990 ("Color Box"), s=w289, f=u32 9678034 ("Color Box")) -> (s? t:f=w283:u32)
          n139 = Bundle(cluster=w306, "Slug"=w304, "Expiration Date"=w299, "Expired?"=w286, "Id"=w285, "active"=FALSE, "Color Box"=w283) -> (w298:T1)
        }
        n140 = Array Size(array=w262) -> (size(s)=w264:i32)
        n141 = Index Array(array=w262) -> (element=w272:T1)  [unwired: 1 in]
        n142 = Greater?(x=w264, y=w265) -> (0:w266:bool)
        n143 = Unbundle By Name(w272) -> ("Id"=w271:i32)
        n144 = Bundle By Name(cluster=w279, "All_Instruments_Cals"=w274, "Slug list All"=w262, "Selected Slug"=w271) -> (w278:T7)
        n145 = Select(t=w265, s=w266, f=w264) -> (s? t:f=w263:i32)
        n146 = property class="Arr (strict)"(reference=w267, error in=w268, "Number of Rows"=w263) -> (error out=w269:errorcluster)  [unwired: 1 out]
        n147 = local write "Slug list"(w262) -> ()
      }
      frame "GetInstruments" {
        n148 = Unbundle By Name(w328) -> ("ByteQXAPIBase in"=w329:refnum<class "ByteQXAPIBase.lvclass">)
        n149 = call "InstrumentsList.vi"("error in (no error)"=w330, "ByteQXAPIBase in"=w329) -> ("error out"=w324:errorcluster, "Array"=w323:T4[], "ByteQXAPIBase out"=w327:refnum<class "ByteQXAPIBase.lvclass">)  [unwired: 7 in]
        n150 = for {
          tunnel: w323 -> [w332] mode=indexing
          tunnel: [w331] -> w322 mode=indexing
          n151 = Unbundle By Name(w332) -> ("slug"=w331:string)
        }
        n152 = Bundle By Name(cluster=w328, "ByteQXAPIBase in"=w327, "All_Instruments"=w323, "Instruments_Slug"=w322) -> (w326:T7)
      }
      frame "GetCalibrations" {
        n153 = Unbundle By Name(w343) -> ("Start Calibration"=w340:refnum<vi>)
        n154 = Unbundle By Name(w357) -> ("ByteQXAPIBase in"=w359:refnum<class "ByteQXAPIBase.lvclass">, "Selected Slug"=w360:i32)
        n155 = call-dynamic "ExecutingCalibration.vi"("error in (no error)"=w358, "calibration_id"=w360, "ByteQXAPIBase in"=w359) -> ("error out"=w354:errorcluster, "calibration data"=w351:T3, "ByteQXAPIBase out"=w355:refnum<class "ByteQXAPIBase.lvclass">)  [unwired: 6 in]
        n156 = call "MisurazioniString.vi"("error in (no error)"=w354, "index"=0, "Calibration data"=w351) -> ("error out"=w334:errorcluster, "index"=w337:i32, "String"=w353:string)  [unwired: 6 in]
        n157 = Unbundle By Name(w351) -> ("controls"=w344:T9)
        n158 = for {
          tunnel: w344 -> [w368] mode=indexing
          tunnel: [w362] -> w341
          stop <- w362 stop-if-true
          n159 = Unbundle By Name(w368) -> ("numero_misure_necessarie"=w367:u16, "numero_misure_effettuate"=w366:u32)
          n160 = Less Or Equal?(x=w367, y=w366) -> (x <= y?=w365:bool)
          n161 = Select(t=FALSE, s=w365, f=TRUE) -> (s? t:f=w362:bool)
        }
        n162 = Build Array(w340) -> (w342:refnum<vi>[])
        n163 = call "DisableControls.vi"("Visible"=w341, "Controls"=w342) -> ()  [unwired: 9 in, 1 out]
        n164 = Index Array(array=w344) -> (element=w347:T10)  [unwired: 1 in]
        n165 = Array Size(array=w344) -> (size(s)=w338:i32)
        n166 = Increment(x=w337) -> (x+1=w336:i32)
        n167 = Unbundle By Name(w347) -> ("numero_misure_effettuate"=w345:u32, "numero_misure_necessarie"=w346:u16)
        n168 = Format Into String(format string="%d/%d", error in=w334, w336, w338) -> (resulting string=w335:string, error out=w333:errorcluster)  [unwired: 1 in]
        n169 = Format Into String(format string="%d/%d", error in=w333, w345, w346) -> (resulting string=w348:string, error out=w350:errorcluster)  [unwired: 1 in]
        n170 = Bundle By Name(cluster=w357, "ByteQXAPIBase in"=w355, "Calibrations"=w351, "Misurazioni"=w353, "Misurazioni index"=w337, "Misurazioni n"=w348, "Misure effettuate"=w345, "Calibrations"=w335) -> (w356:T7)
      }
      frame "CheckTotalMisurations" {
        n171 = Unbundle By Name(w375) -> ()  [unwired: 1 out]
        n172 = Unbundle By Name(w372) -> ("Calibrations"=w381:T3, "Cal Index"=w370:i32, "Misure effettuate"=w369:i32)
        n173 = Unbundle By Name(w381) -> ("controls"=w380:T9)
        n174 = Index Array(array=w380, index=w370) -> (element=w379:T10)
        n175 = Unbundle By Name(w379) -> ("numero_misure_necessarie"=w378:u16)
        n176 = Less Or Equal?(x=w378, y=w369) -> (x <= y?=w377:bool)
        n177 = case shown="True" w377 {
          tunnel: [CalibrationStates."StartCalibration" w393] -> w376
          tunnel: w374 -> [w383 w402]
          tunnel: [w383 w388] -> w373
          tunnel: w372 -> [w382 w404]
          tunnel: [w382 w399] -> w371
          tunnel: w370 -> [_ _]
          frame False {
          }
          frame True {
            n178 = Unbundle By Name(w404) -> ("Misure effettuate"=w406:i32, "Cal Index"=w397:i32, "Waveform Chart"=w401:refnum<vi>, "Calibrations"=w410:T3)
            n179 = Unbundle By Name(w410) -> ("controls"=w398:T9)
            n180 = Index Array(array=w398, index=w397) -> (element=w409:T10)
            n181 = Unbundle By Name(w409) -> ("numero_misure_necessarie"=w408:u16)
            n182 = property class="WFChart (strict)"(reference=w401, error in=w402, "History Data"=dbl[] []) -> (error out=w400:errorcluster)  [unwired: 1 out]
            n183 = Less Or Equal?(x=w408, y=w406) -> (x <= y?=w407:bool)
            n184 = case shown="True" w407 {
              tunnel: w397 -> [w416 w421]
              tunnel: [w416 w420] -> w414
              tunnel: w406 -> [w415 _]
              tunnel: [w415 w417] -> w405
              tunnel: w398 -> [_ w419]
              frame False {
              }
              frame True {
                n185 = Increment(x=w421) -> (x+1=w420:i32)
                n186 = Index Array(array=w419, index=w420) -> (element=w418:T10)
                n187 = Unbundle By Name(w418) -> ("numero_misure_effettuate"=w417:u32)
              }
            }
            n188 = Array Size(array=w398) -> (size(s)=w385:i32)
            n189 = Decrement(x=w385) -> (x-1=w392:i32)
            n190 = call "MisurazioniString.vi"("error in (no error)"=w400, "index"=w414, "Calibration data"=w410) -> ("error out"=w389:errorcluster, "index"=w386:i32, "String"=w413:string)  [unwired: 6 in]
            n191 = Less Or Equal?(x=w392, y=w397) -> (x <= y?=w396:bool)
            n192 = Increment(x=w386) -> (x+1=w390:i32)
            n193 = Format Into String(format string="%d/%d", error in=w389, w390, w385) -> (resulting string=w387:string, error out=w388:errorcluster)  [unwired: 1 in]
            n194 = Bundle By Name(cluster=w404, "Misure effettuate"=w405, "Cal Index"=w414, "Misurazioni"=w413, "Misurazioni index"=w386, "Id Failed"=u32 0, "Failed?"=FALSE, "Calibrations"=w387) -> (w399:T7)
            n195 = Select(t=CalibrationStates."AllowApprove", s=w396, f=CalibrationStates."CheckTotalMisurations") -> (s? t:f=w393:T2)
          }
        }
      }
      frame "StartCalibration" {
        n196 = Unbundle By Name(w437) -> ("Outcome"=w436:refnum<vi>, "Avanti"=w425:refnum<vi>, "Repeat"=w422:refnum<vi>)
        n197 = property class="Str"(reference=w436, error in=w433, "Text.BGColor"=u32 9678034 ("Text.Text Colors:BG Color")) -> (error out=w434:errorcluster)  [unwired: 1 out]
        n198 = Build Array(w425, w422) -> (w427:refnum<vi>[])
        n199 = Unbundle By Name(w448) -> ("Calibrations"=w452:T3, "New Val"=w445:dbl, "Cal Index"=w432:i32, "Misure effettuate"=w429:i32)  [unwired: 1 out]
        n200 = call "DisableControls.vi"("Visible"=FALSE, "Controls"=w427) -> ()  [unwired: 9 in, 1 out]
        n201 = Unbundle By Name(w452) -> ("controls"=w424:T9)
        n202 = call "FGVTimer.vi"("error in"=w434) -> ("error out"=w441:errorcluster, "Elapsed?"=w449:bool)  [unwired: 8 in, 1 out]
        n203 = Index Array(array=w424, index=w432) -> (element=w451:T10)
        n204 = Unbundle By Name(w451) -> ("riferimento_obiettivo"=w443:dbl)
        "Reference value" <- w443
        n205 = Index Array(array=w424, index=w432) -> (element=w431:T10)
        n206 = Unbundle By Name(w431) -> ("numero_misure_necessarie"=w430:u16)
        n207 = case shown="False" w449 {
          tunnel: w443 -> [w459 _]
          tunnel: [CalibrationStates."StartCalibration" CalibrationStates."ManageCalibration"] -> w446
          tunnel: [w453 w462] -> w444
          tunnel: w445 -> [_ w462]
          frame False {
            n208 = Quotient & Remainder(x=w459, y=10.0) -> (floor(x/y)=w458:dbl)  [unwired: 1 out]
            n209 = Add(x=w459, y=w458) -> (x+y=w457:dbl)
            n210 = Subtract(x=w459, y=w458) -> (x-y=w454:dbl)
            n211 = To Quad Integer(1:w457) -> (0:w456:i64)
            n212 = To Quad Integer(1:w454) -> (0:w455:i64)
            n213 = call-poly <vilib>:"Random Number (Range).vi"("lower bound (-100)"=w455, "upper bound (100)"=w456) -> ("number"=w453:i64)  [unwired: 9 in]
            "Waveform Chart" <- w453
          }
          frame True {
          }
        }
        "Measured value" <- w444
        n214 = Increment(x=w429) -> (x+1=w428:i32)
        n215 = Format Into String(format string="%d/%d", error in=w441, w428, w430) -> (resulting string=w440:string, error out=w423:errorcluster)  [unwired: 1 in]
        n216 = Bundle By Name(cluster=w448, "Next State"=w446, "New Val"=w444, "Misurazioni n"=w440, "Stato"="Executing calibration", "Esito"="...") -> (w447:T7)
      }
      frame "ManageCalibration" {
        n217 = Unbundle By Name(w484) -> ("ByteQXAPIBase in"=w487:refnum<class "ByteQXAPIBase.lvclass">, "Calibrations.controls"=w490:T9, "New Val"=w486:dbl, "Id Failed"=w482:u32, "Failed?"=w480:bool, "Cal Index"=w470:i32, "Misure effettuate"=w468:i32)
        n218 = Unbundle By Name(w477) -> ("Repeat"=w466:refnum<vi>, "Avanti"=w467:refnum<vi>, "Outcome"=w474:refnum<vi>)
        n219 = Index Array(array=w490, index=w470) -> (element=w489:T10)
        n220 = Unbundle By Name(w489) -> ("id"=w488:u16, "riferimento_obiettivo"=w485:dbl)
        n221 = disable-structure shown="Enabled" {
          disable-tunnel: w488 -> [w526 _]
          disable-tunnel: w487 -> [w525 w546]
          disable-tunnel: w486 -> [w524 w548]
          disable-tunnel: w485 -> [w523 w549]
          disable-tunnel: w471 -> [w522 w547]
          disable-tunnel: [w518 w547] -> w473
          disable-tunnel: w482 -> [w521 _]
          disable-tunnel: [w517 w546] -> w481
          disable-tunnel: w480 -> [w520 _]
          disable-tunnel: [w519 w544] -> w469
          disable-tunnel: [w514 _] -> w464
          frame Enabled {
            n222 = case shown="False" w520 {
              tunnel: w525 -> [w534 w543]
              tunnel: w523 -> [w533 w536]
              tunnel: w524 -> [w532 w541]
              tunnel: w522 -> [w531 w542]
              tunnel: [w530 w539] -> w518
              tunnel: w526 -> [w528 w538]
              tunnel: [w529 w540] -> w517
              tunnel: [w528 w538] -> _
              tunnel: w521 -> [_ w537]
              tunnel: [w527 w535] -> w516
              frame False {
                n223 = call-dynamic "AddMeasurement.vi"("measurement-group-id"=w528, "error in (no error)"=w531, "instrument measure"=w532, "reference measure"=w533, "ByteQXAPIBase in"=w534) -> ("error out"=w530:errorcluster, "measurement data"=w527:T11, "ByteQXAPIBase out"=w529:refnum<class "ByteQXAPIBase.lvclass">)  [unwired: 4 in]
              }
              frame True {
                n224 = call-dynamic "EditMeasurement.vi"("reference measure"=w536, "error in (no error)"=w542, "instrument measure"=w541, "measurement-id"=w537, "ByteQXAPIBase in"=w543) -> ("error out"=w539:errorcluster, "measurement data"=w535:T11, "ByteQXAPIBase out"=w540:refnum<class "ByteQXAPIBase.lvclass">)  [unwired: 4 in]
              }
            }
            n225 = Unbundle By Name(w516) -> ("id"=w514:i32, "is_correct"=w515:bool)
            n226 = Not(x=w515) -> (.not. x?=w519:bool)
          }
          frame Disabled {
            n227 = Equal?(x=w549, y=w548) -> (x = y?=w545:bool)
            n228 = Not(x=w545) -> (.not. x?=w544:bool)
          }
        }
        n229 = case shown="True" w469 {
          tunnel: ["PASSED" ("Esito") "FAILED" ("Esito")] -> w475
          tunnel: w474 -> [w507 w511]
          tunnel: w473 -> [w505 w510]
          tunnel: [w504 w509] -> w472
          frame False {
            n230 = property class="Str"(reference=w507, error in=w505, "Text.BGColor"=u32 5558784 ("Text.Text Colors:BG Color")) -> (error out=w504:errorcluster)  [unwired: 1 out]
          }
          frame True {
            n231 = property class="Str"(reference=w511, error in=w510, "Text.BGColor"=u32 16737380 ("Text.Text Colors:BG Color")) -> (error out=w509:errorcluster)  [unwired: 1 out]
          }
        }
        n232 = case shown="True" w469 {
          tunnel: w468 -> [w498 w503]
          tunnel: [w497 w503] -> w465
          tunnel: w466 -> [w492 w500]
          tunnel: w467 -> [w491 w499]
          frame False {
            n233 = Build Array(w491) -> (w494:refnum<vi>[])
            n234 = Build Array(w492) -> (w496:refnum<vi>[])
            n235 = Increment(x=w498) -> (x+1=w497:i32)
            n236 = call "DisableControls.vi"("Visible"=FALSE, "Controls"=w496) -> ()  [unwired: 9 in, 1 out]
            n237 = call "DisableControls.vi"("Visible"=TRUE, "Controls"=w494) -> ()  [unwired: 9 in, 1 out]
          }
          frame True {
            n238 = Build Array(w500, w499) -> (w502:refnum<vi>[])
            n239 = call "DisableControls.vi"("Visible"=TRUE, "Controls"=w502) -> ()  [unwired: 9 in, 1 out]
          }
        }
        n240 = Bundle By Name(cluster=w484, "ByteQXAPIBase in"=w481, "Id Failed"=w464, "Failed?"=w469, "Next State"=CalibrationStates."Idle", "Stato"="Calibration executed", "Esito"=w475, "Misure effettuate"=w465) -> (w483:T7)
      }
      frame "AllowApprove" {
        n241 = Unbundle By Name(w559) -> ("Repeat"=w558:refnum<vi>, "Approvation"=w556:refnum<vi>, "Avanti"=w557:refnum<vi>)
        n242 = Unbundle By Name(w550) -> ("Calibrations.controls"=w551:T9, "Misure effettuate"=w555:i32, "Cal Index"=w554:i32)
        n243 = Array Size(array=w551) -> (size(s)=w566:i32)
        n244 = Decrement(x=w566) -> (x-1=w565:i32)
        n245 = Index Array(array=w551, index=w554) -> (element=w564:T10)
        n246 = Less Or Equal?(x=w565, y=w554) -> (x <= y?=w561:bool)
        n247 = Unbundle By Name(w564) -> ("numero_misure_necessarie"=w563:u16)
        n248 = Equal?(x=w555, y=w563) -> (x = y?=w562:bool)
        n249 = And(x=w562, y=w561) -> (x .and. y?=w560:bool)
        n250 = case shown="True" w560 {
          tunnel: w556 -> [_ w570]
          tunnel: w557 -> [_ w573]
          tunnel: w558 -> [_ w567]
          frame False {
          }
          frame True {
            n251 = Build Array(w570) -> (w569:refnum<vi>[])
            n252 = Build Array(w573, w567) -> (w572:refnum<vi>[])
            n253 = call "DisableControls.vi"("Visible"=TRUE, "Controls"=w569) -> ()  [unwired: 9 in, 1 out]
            n254 = call "DisableControls.vi"("Visible"=FALSE, "Controls"=w572) -> ()  [unwired: 9 in, 1 out]
          }
        }
      }
      frame "Approve" {
        n255 = Unbundle By Name(w584) -> ("Cancel"=w574:refnum<vi>, "Approvation"=w583:refnum<vi>)
        n256 = Build Array(w583) -> (w582:refnum<vi>[])
        n257 = call "DisableControls.vi"("Visible"=FALSE, "Controls"=w582) -> ()  [unwired: 9 in, 1 out]
        n258 = disable-structure shown="Enabled" {
          disable-tunnel: w587 -> [w588 w599]
          disable-tunnel: w586 -> [w591 w598]
          disable-tunnel: [w590 w599] -> w580
          disable-tunnel: [w589 w598] -> w576
          frame Enabled {
            n259 = in-place {
              in-place-border: w588 -> [w595]
              in-place-border: [w594] -> w589
              in-place-border: w591 -> [w592]
              n260 = in-place-cluster #2(w588) -> ("ByteQXAPIBase in"=w597:refnum<class "ByteQXAPIBase.lvclass">)
              n261 = Unbundle By Name(w595) -> ("Selected Slug"=w593:i32)
              n262 = call-dynamic "SendRequestApproval.vi"("error in (no error)"=w592, "calibration-id"=w593, "ByteQXAPIBase in"=w597) -> ("error out"=w594:errorcluster, "ByteQXAPIBase out"=w596:refnum<class "ByteQXAPIBase.lvclass">)  [unwired: 6 in, 1 out]
              n263 = in-place-cluster #2("ByteQXAPIBase in"=w596) -> (w590:T7)
            }
          }
          frame Disabled {
          }
        }
        n264 = property class="Bool"(reference=w574, error in=w576, "BoolText.Text"="RESTART" ("Boolean Text.Text")) -> (error out=w575:errorcluster)  [unwired: 1 out]
        n265 = Bundle By Name(cluster=w580, "Stato"="Request of approval sent") -> (w579:T7)
      }
    }
    n266 = Unbundle By Name(w43) -> ("Misurazioni"=→"Calibration n.":string, "Misurazioni n"=→"Calibration n.":string, "Stato"=→"Status":string, "Esito"=→"Outcome":string, "Calibrations"=→"Calibrations":string)
    n267 = Or(x=w34, y=w35) -> (x .or. y?=w36:bool)
  }
  n268 = call <vilib>:"Simple Error Handler.vi"("error in (no error)"=w1) -> ()  [unwired: 4 in, 5 out]
